vi "FocusOnThisItem.vi"(8 "error in (no error)":errorcluster, 9 "Focus?(False)":bool, 10 "ItemCtlRef":refnum<vi>, 11 "TableItem in":refnum<class "TableItem.lvclass">) -> (0 "error out":errorcluster, 3 "TableItem out":refnum<class "TableItem.lvclass">)   [LabVIEW 2015, in "ActorManagement.lvlib" / "TableItem.lvclass"]
uses:
  TableItem.lvclass
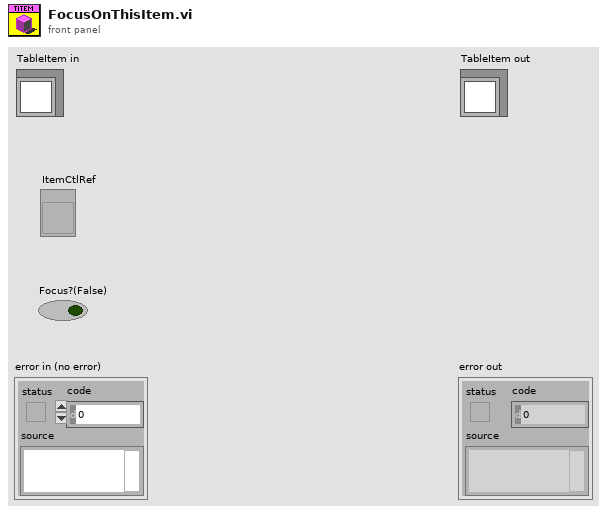
[diagram p1: front panel]
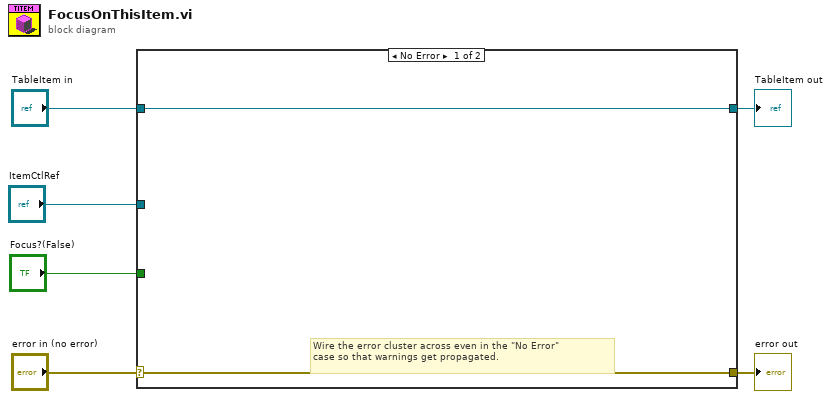
[diagram p0: block diagram]
diagram:
  n1 = case shown="No Error" "error in (no error)" {
    selector: "error in (no error)" -> [w7 w10]
    tunnel: [w7 w10] -> w5
    tunnel: [w8 w9] -> w3
    tunnel: "TableItem in" -> [w8 w9]
    tunnel: "ItemCtlRef" -> [_ _]
    tunnel: "Focus?(False)" -> [_ _]
    frame No Error {
      # "Wire the error cluster across even in the \"No Error\"\ncase so that warnings get propagated."
    }
    frame Error {
    }
  }
  "error out" <- w5
  "TableItem out" <- w3
